vi "resolve fpga references.vi"(0 "data to unwrap":string) -> (4 "remaining string":string, 6 "ResourceName":string, 8 "Bitfile path":path, 10 "Bitfile Exe Dir":path)   [LabVIEW 2014, in "io configuration.lvclass"]
uses:
  io configuration.lvclass
  <vilib>/NI/Configuration Framework/serializable configuration/NISE_CEF_serializable configuration.lvclass
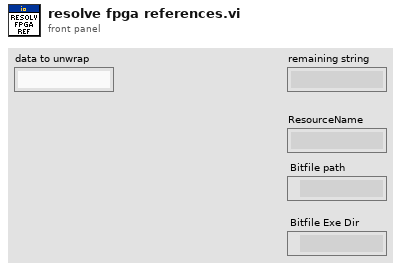
[diagram p1: front panel]
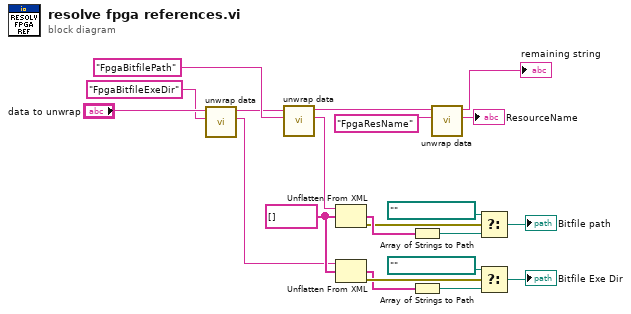
[diagram p0: block diagram]
diagram:
  w2 = string[] [] ("array of strings")
  n1 = call <vilib>:"unwrap data.vi"("identifier"="FpgaBitfileExeDir" ("additional identifier"), "data to unwrap"="data to unwrap") -> ("unwrapped data"=w1:string, "remaining string"=w10:string)  [unwired: 8 in]
  n2 = call <vilib>:"unwrap data.vi"("identifier"="FpgaBitfilePath" ("additional identifier"), "data to unwrap"=w10) -> ("unwrapped data"=w18:string, "remaining string"=w20:string)  [unwired: 8 in]
  n3 = Unflatten From XML(xml string=w18, type=w2) -> (value=w17:string[], error out=w13:errorcluster)  [unwired: 1 in]
  n4 = Unflatten From XML(xml string=w1, type=w2) -> (value=w3:string[], error out=w6:errorcluster)  [unwired: 1 in]
  n5 = Array of Strings to Path(0:w17) -> (2:w14:path)  [unwired: 1 in]
  n6 = Array of Strings to Path(0:w3) -> (2:w5:path)  [unwired: 1 in]
  n7 = call <vilib>:"unwrap data.vi"("identifier"="FpgaResName" ("additional identifier"), "data to unwrap"=w20) -> ("unwrapped data"=→"ResourceName":string, "remaining string"=→"remaining string":string)  [unwired: 8 in]
  n8 = Select(t=path "", s=w13, f=w14) -> (s? t:f=→"Bitfile path":path)
  n9 = Select(t=path "", s=w6, f=w5) -> (s? t:f=→"Bitfile Exe Dir":path)
